vi "Configure Multi Eval Meas List Segment CC Center Frequency.vi"(6 "Center Frequency (1.95GHz)":dbl=1950000000.0 format="%#.9p", 7 "CC (1)":T1=1, 8 "error in (no error)":errorcluster, 9 "Segment (1)":i32=1, 10 "Instance (1)":T2=1, 11 "VISA resource name":refnum<visa-resource-name>) -> (0 "error out":errorcluster, 3 "VISA resource name out":refnum<visa-resource-name>)   [LabVIEW 2020, in "Rohde&Schwarz CMWXP NR FR1 Measurement.lvlib"]
doc: "Selects the center frequency of carrier <cc>, used in segment <no>.\n\nAttribute:\nRSCMWXPNRFR1M_ATTR_MULTI_EVAL_MEAS_LIST_SEGMENT_CC_CENTER_FREQUENCY\n\nRemote-control command:\nCONFigure:NRSub:MEAS<i>:LIST:SEGMent<no>[:CC<cc>]:FREQuency"
uses:
  <instrlib>/Rohde&Schwarz CMWXP NR FR1 Measurement/Rohde&Schwarz CMWXP NR FR1 Measurement.lvlib
  <instrlib>/Rohde&Schwarz CMWXP NR FR1 Measurement/Private/_Instance.ctl
  <instrlib>/Rohde&Schwarz CMWXP NR FR1 Measurement/Private/_Carrier Component.ctl
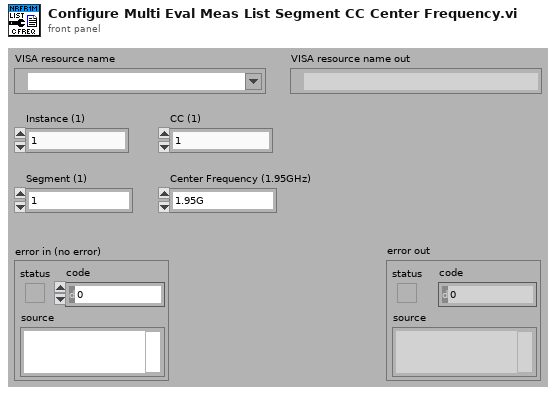
[diagram p1: front panel]
types:
  T1 = typedef "Rohde&Schwarz CMWXP NR FR1 Measurement.lvlib/_Carrier Component.ctl" = i32
  T2 = typedef "Rohde&Schwarz CMWXP NR FR1 Measurement.lvlib/_Instance.ctl" = i32
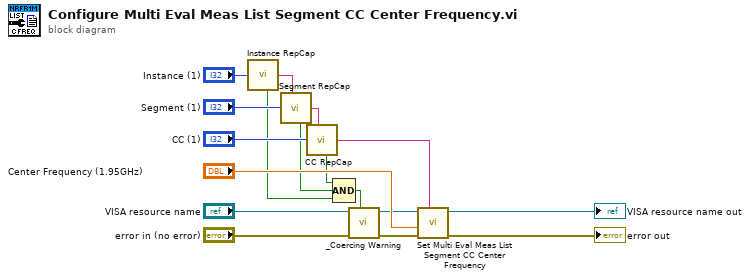
[diagram p0: block diagram]
diagram:
  n1 = call <instrlib>:"Instance RepCap.vi"("Instance In"="Instance (1)") -> ("In Range?"=w3:bool, "RepCap Identifier Out"=w12:string)  [unwired: 1 in]
  n2 = call <instrlib>:"Segment RepCap.vi"("Segment In"="Segment (1)", "RepCap String In (\"\")"=w12) -> ("In Range?"=w2:bool, "RepCap Identifier Out"=w10:string)
  n3 = call <instrlib>:"CC RepCap.vi"("CC In"="CC (1)", "RepCap String In (\"\")"=w10) -> ("In Range?"=w1:bool, "RepCap Identifier Out"=w9:string)
  n4 = Compound Arithmetic op=AND(w1, w2, w3) -> (w4:bool)
  n5 = call <instrlib>:"_Coercing Warning.vi"("In Range?"=w4, "error in (no error)"="error in (no error)", "VISA resource name"="VISA resource name") -> ("error out"=w6:errorcluster, "VISA resource name out"=w5:refnum<visa-resource-name>)  [unwired: 7 in]
  n6 = call "Set Multi Eval Meas List Segment CC Center Frequency"("Repeated Capabilities"=w9, "error in (no error)"=w6, "Multi Eval Meas List Segment CC Center Frequency (0.0)"="Center Frequency (1.95GHz)", "instrument handle"=w5) -> ("error out"=→"error out":errorcluster, "instrument handle out"=→"VISA resource name out":refnum<visa-resource-name>)  [unwired: 6 in]
